vi "Fetch Multi Eval Meas List IEM Margin RB Index Results.vi"(8 "error in (no error)":errorcluster, 9 "Result Type (Current)":i32(ring) items=["Current"=0, "Extreme"=2], 10 "Instance (1)":T2=1, 11 "VISA resource name":refnum<visa-resource-name>) -> (0 "error out":errorcluster, 1 "IEM Margin RB Index Results":T1(array[cluster]), 2 "Reliability":i32, 3 "VISA resource name out":refnum<visa-resource-name>)   [LabVIEW 2020, in "Rohde&Schwarz CMXP NR FR2 Measurement.lvlib"]
doc: "Returns resource block indices of the inband emission measurement for all measured list mode segments.\n\nAttributes:\nRSCMXPNRFR2M_ATTR_FETCH_MULTI_EVAL_MEASUREMENT_LIST_IEM_MARGIN_RB_INDEX_CURRENT_RESULTS\nRSCMXPNRFR2M_ATTR_FETCH_MULTI_EVAL_MEASUREMENT_LIST_IEM_MARGIN_RB_INDEX_EXTREME_RESULTS\n\nRemote-control commands:\nFETCh:NRMMw:MEAS<i>:MEValuation:LIST:IEMission:MARGin:RBINdex:CURRent?\nFETCh:NRMMw:MEAS<i>:MEValuation:LIST:IEMission:MARGin:RBINdex:EXTReme?"
uses:
  <instrlib>/Rohde&Schwarz CMXP NR FR2 Measurement/Rohde&Schwarz CMXP NR FR2 Measurement.lvlib
  <instrlib>/Rohde&Schwarz CMXP NR FR2 Measurement/Private/_Instance.ctl
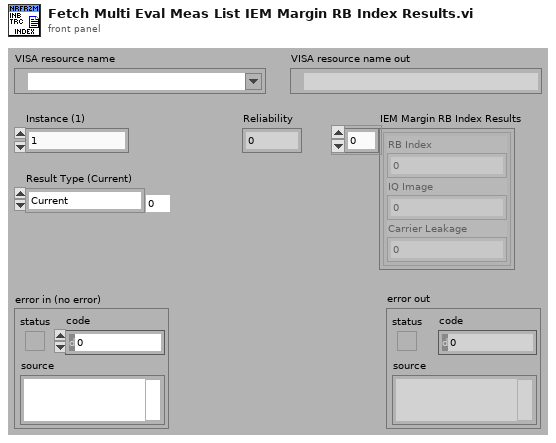
[diagram p1: front panel]
types:
  T1 = cluster{"RB Index":i32, "IQ Image":i32, "Carrier Leakage":i32}[]
  T2 = typedef "Rohde&Schwarz CMXP NR FR2 Measurement.lvlib/_Instance.ctl" = i32
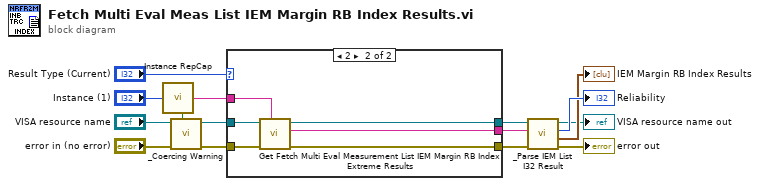
[diagram p0: block diagram]
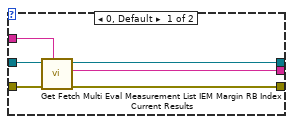
[diagram p2: hidden frame]
diagram:
  n1 = call <instrlib>:"Instance RepCap.vi"("Instance In"="Instance (1)") -> ("In Range?"=w13:bool, "RepCap Identifier Out"=w10:string)  [unwired: 1 in]
  n2 = call <instrlib>:"_Coercing Warning.vi"("In Range?"=w13, "error in (no error)"="error in (no error)", "VISA resource name"="VISA resource name") -> ("error out"=w12:errorcluster, "VISA resource name out"=w11:refnum<visa-resource-name>)  [unwired: 7 in]
  n3 = case shown="2" "Result Type (Current)" {
    tunnel: w12 -> [w21 w27]
    tunnel: w11 -> [w20 w26]
    tunnel: w10 -> [w19 w25]
    tunnel: [w18 w24] -> w9
    tunnel: [w17 w23] -> w7
    tunnel: [w16 w22] -> w6
    frame 0, Default {
      n4 = call "Get Fetch Multi Eval Measurement List IEM Margin RB Index Current Results"("Repeated Capabilities"=w19, "error in (no error)"=w21, "instrument handle"=w20) -> ("error out"=w18:errorcluster, "Fetch Multi Eval Measurement List IEM Margin RB Index Current Results"=w17:string, "instrument handle out"=w16:refnum<visa-resource-name>)  [unwired: 6 in]
    }
    frame 2 {
      n5 = call "Get Fetch Multi Eval Measurement List IEM Margin RB Index Extreme Results"("Repeated Capabilities"=w25, "error in (no error)"=w27, "instrument handle"=w26) -> ("error out"=w24:errorcluster, "Fetch Multi Eval Measurement List IEM Margin RB Index Extreme Results"=w23:string, "instrument handle out"=w22:refnum<visa-resource-name>)  [unwired: 6 in]
    }
  }
  n6 = call <instrlib>:"_Parse IEM List I32 Result.vi"("error in (no error)"=w9, "Input String"=w7, "VISA resource name"=w6) -> ("error out"=→"error out":errorcluster, "Results"=→"IEM Margin RB Index Results":T1, "Reliability"=→"Reliability":i32, "VISA resource name out"=→"VISA resource name out":refnum<visa-resource-name>)  [unwired: 5 in]
